vi "Edge Detect Column (SubVI).vi"(10 "Pixel In":u8, 11 "Column #":u16) -> (3 "Pixel Out":u8)   [LabVIEW 2015]
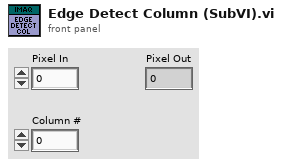
[diagram p1: front panel]
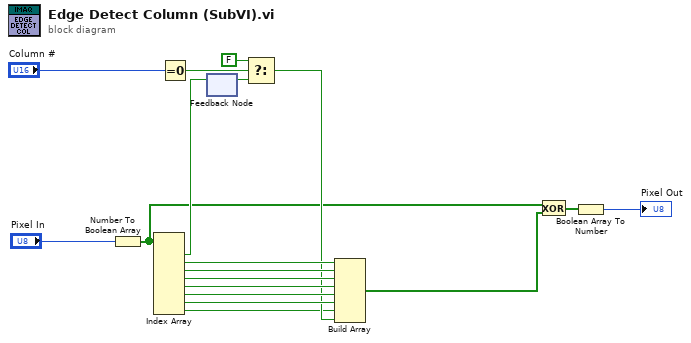
[diagram p0: block diagram]
diagram:
  n1 = Number To Boolean Array(number="Pixel In") -> (Boolean array=w6:bool[])
  n2 = Index Array(array=w6) -> (element #1=w7:bool, element #2=w16:bool, element #3=w15:bool, element #4=w14:bool, element #5=w13:bool, element #6=w12:bool, element #7=w11:bool, element #8=w8:bool)  [unwired: 8 in]
  n3 = Equal To 0?(x="Column #") -> (x = 0?=w18:bool)
  n4 = feedback #1() -> (w1:bool)  [unwired: 1 in]
  n5 = feedback-in #1(w7) -> ()
  n6 = Select(t=FALSE ("f"), s=w18, f=w1) -> (s? t:f=w9:bool)
  n7 = Build Array(w16, w15, w14, w13, w12, w11, w8, w9) -> (w10:bool[])
  n8 = Exclusive Or(1:w10, 2:w6) -> (0:w3:bool[])
  n9 = Boolean Array To Number(Boolean array=w3) -> (number=→"Pixel Out":u8)
